vi "UPDATE FROM DB.vi"(8 "error in":errorcluster, 10 "object":refnum<class "_ISerializable.lvclass">, 11 "orm in":refnum<class "LV-ORM.lvclass">) -> (0 "error out":errorcluster, 3 "orm out":refnum<class "LV-ORM.lvclass">)   [LabVIEW 2018, in "LV-ORM.lvclass"]
uses:
  LV-ORM.lvclass
  _Serializable Base Object/_ISerializable.lvclass
  <userlib>/_OpenG.lib/array/array.llb/Filter 1D Array (String)__ogtk.vi
  <userlib>/_OpenG.lib/array/array.llb/Delete Elements from 1D Array (String)__ogtk.vi
  Serializer/Serializer.lvclass
panel:
  out "column names":string[](array[string])
  out "names":string[](array[string])
  out "recordset data":variant[][](array[variant])
  out "x != y?":bool[](array[boolean])
  out "update query":string
  out "select query":string
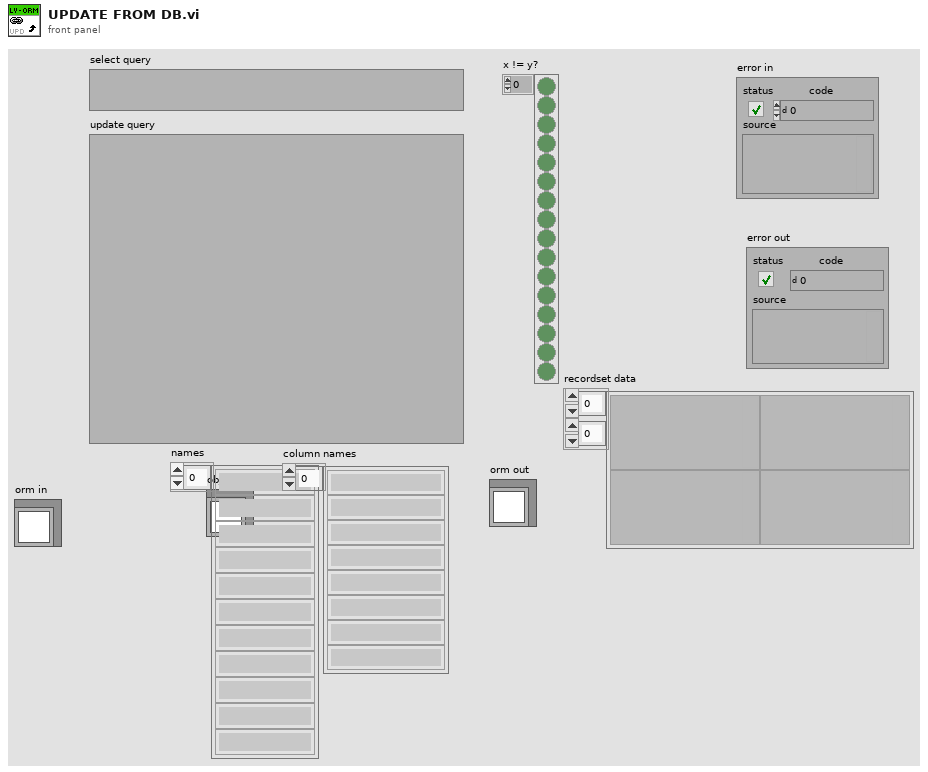
[diagram p1: front panel]
types:
  T1 = typedef "key-value-type cluster.ctl" = cluster{"names":string[], "values":string[], "type":string[], "class name":string}
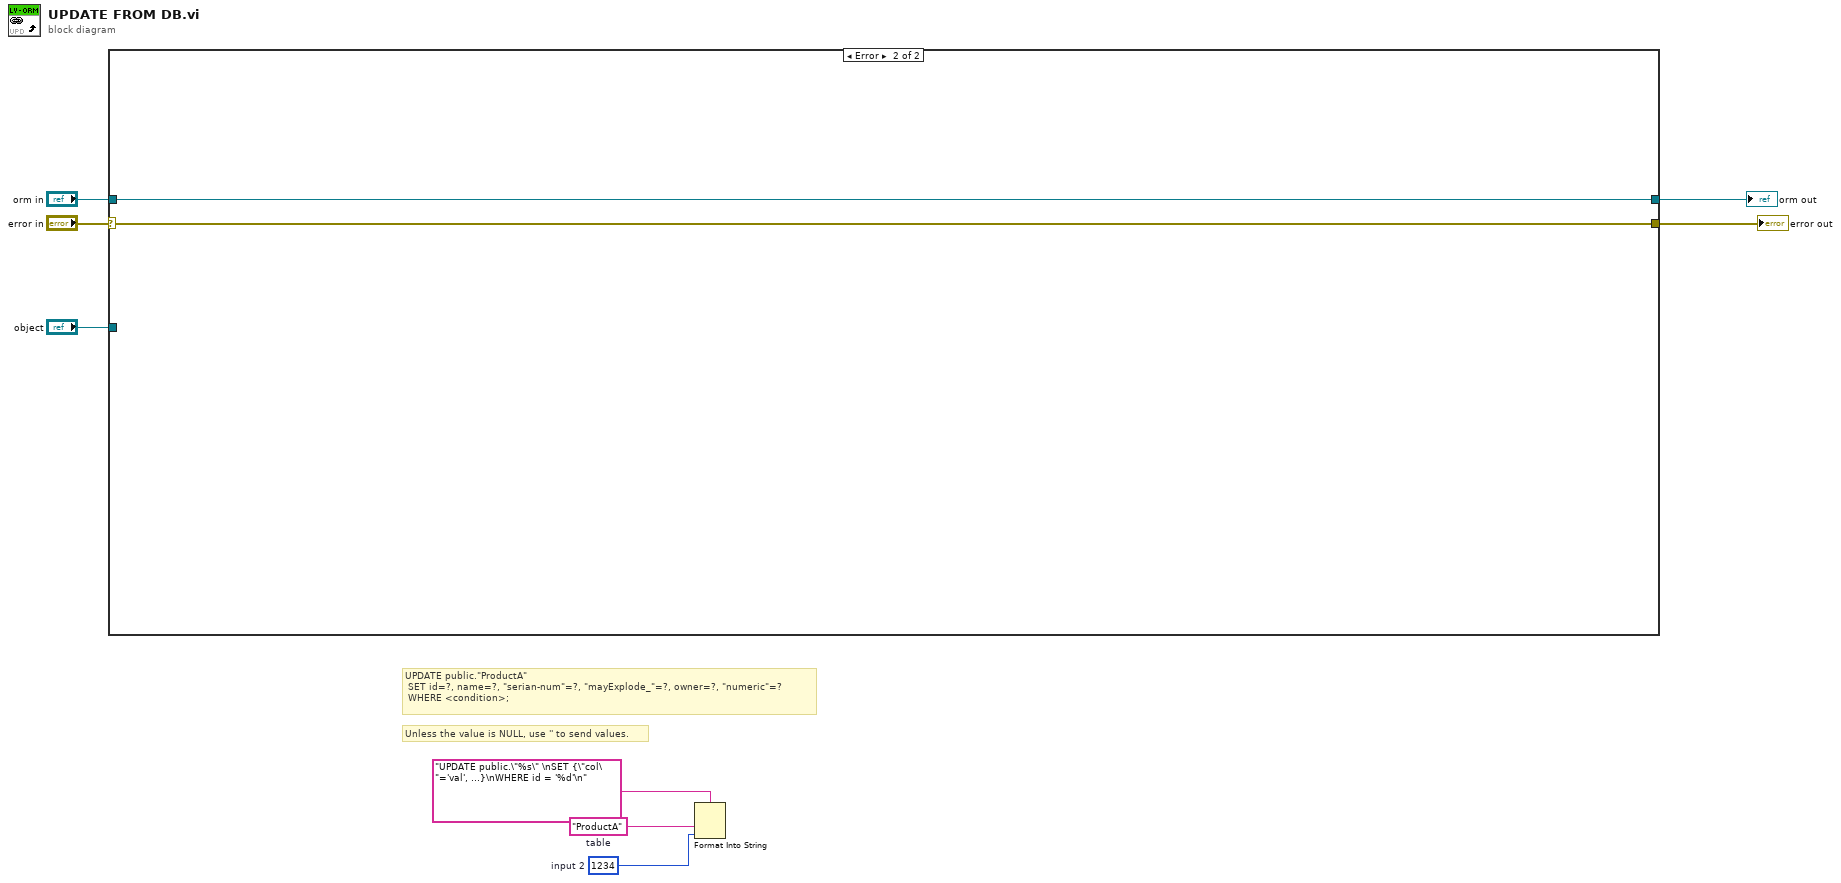
[diagram p0: block diagram]
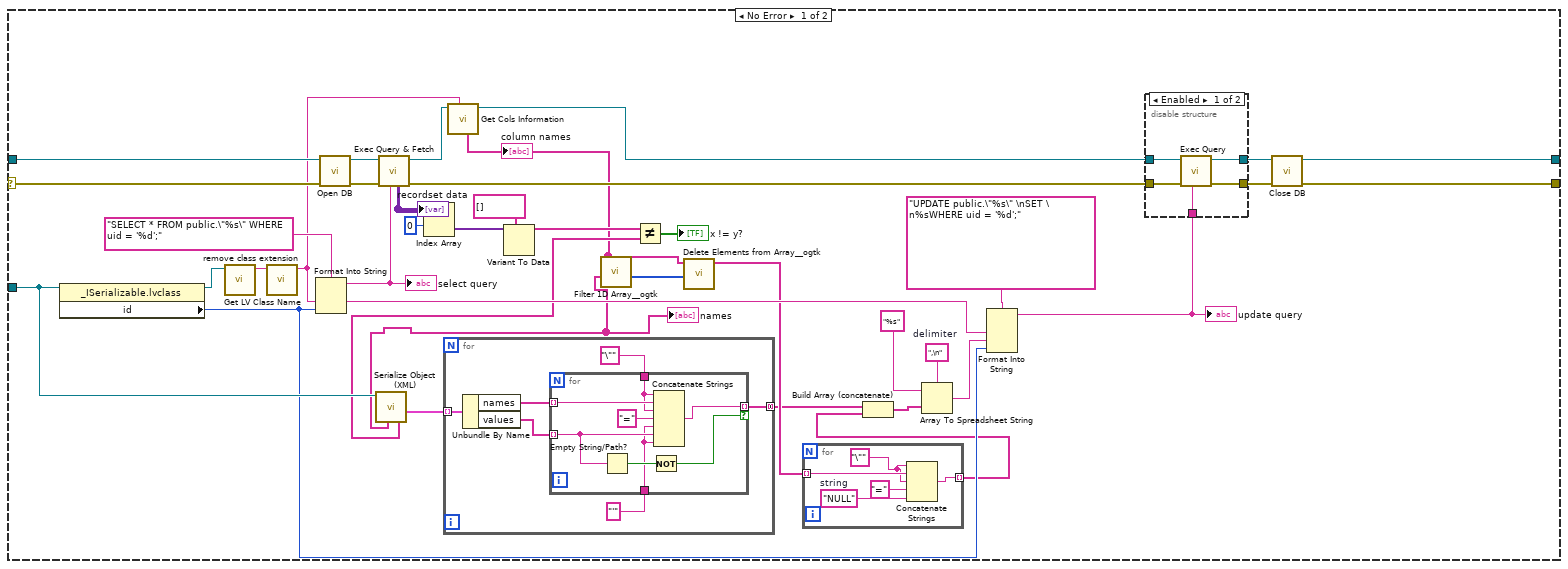
[diagram p2: hidden frame]
diagram:
  w1 = 1234  # input 2
  w2 = "ProductA"  # table
  # "Unless the value is NULL, use '' to send values."
  # "UPDATE public.\"ProductA\"\n\tSET id=?, name=?, \"serian-num\"=?, \"mayExplode_\"=?, owner=?, \"numeric\"=?\n\tWHERE <condition>;"
  n1 = case shown="Error" "error in" {
    selector: "error in" -> [w33 w74]
    tunnel: [w26 w74] -> w7
    tunnel: [w43 w73] -> w6
    tunnel: "orm in" -> [w42 w73]
    tunnel: "object" -> [w37 _]
    frame No Error {
      w30 = ",\n"  # delimiter
      n2 = property class="_ISerializable.lvclass"(reference=w37) -> (reference out=w39:refnum<class "_ISerializable.lvclass">, "id"=w27:i32)  [unwired: 1 in, 1 out]
      n3 = call <vilib>:"Get LV Class Name.vi"("object"=w39) -> ("class name"=w40:string)  [unwired: 9 in, 1 out]
      n4 = call "remove class extension.vi"("class name in"=w40) -> ("class name out"=w18:string)  [unwired: 10 in]
      n5 = Format Into String(format string="SELECT * FROM public.\"%s\" WHERE uid = '%d';", w18, w27) -> (resulting string=w13:string)  [unwired: 2 in, 1 out]
      "select query" <- w13
      n6 = call "Open DB.vi"("error in (no error)"=w33, "LV-ORM in"=w42) -> ("error out"=w38:errorcluster, "LV-ORM out"=w41:refnum<class "LV-ORM.lvclass">)  [unwired: 8 in]
      n7 = call "Serialize Object (XML).vi"("object in"=w37) -> ("key-value-type"=w29:T1[], "values"=w16:string[], "names"=w9:string[])  [unwired: 6 in, 2 out]
      "names" <- w9
      n8 = call "Exec Query & Fetch.vi"("scripts"=w13, "error in"=w38, "orm in"=w41) -> ("error out"=w34:errorcluster, "orm out"=w20:refnum<class "LV-ORM.lvclass">, "recordset data"=w36:variant[][])  [unwired: 6 in]
      "recordset data" <- w36
      n9 = Index Array(array=w36, index (row)=0) -> (element=w32:variant[])  [unwired: 1 in]
      n10 = for {
        tunnel: w29 -> [w57] mode=indexing
        tunnel: [w56] -> w12 mode=concatenating
        n11 = Unbundle By Name(w57) -> ("names"=w55:string[], "values"=w53:string[])
        n12 = for {
          tunnel: w55 -> [w65] mode=indexing
          tunnel: [w64] -> w56 mode=indexing if=w59
          tunnel: "\"" -> [w63]
          tunnel: w53 -> [w61] mode=indexing
          tunnel: "'" -> [w58]
          n13 = Empty String/Path?(string/path=w61) -> (empty?=w60:bool)
          n14 = Not(x=w60) -> (.not. x?=w59:bool)
          n15 = Concatenate Strings(w63, w65, w63, "=", w58, w61, w58) -> (w64:string)
        }
      }
      n16 = call "Get Cols Information.vi"("Table Name"=w18, "LV-ORM in"=w20) -> ("LV-ORM out"=w19:refnum<class "LV-ORM.lvclass">, "column names"=w15:string[])  [unwired: 5 in, 3 out]
      "column names" <- w15
      n17 = Variant To Data(type=string[] [], Variant=w32) -> (data=w22:string[])  [unwired: 1 in, 1 out]
      n18 = call-poly <userlib>:"Filter 1D Array__ogtk.vi"("items to filter"=w9, "array"=w15) -> ("filtered item indices"=w14:i32[])  [unwired: 4 in, 1 out]
      n19 = Not Equal?(x=w22, y=w16) -> (x != y?=→"x != y?":bool[])
      n20 = call-poly <userlib>:"Delete Elements from Array__ogtk.vi"("indices"=w14, "array"=w15) -> ("array w/ subset deleted"=w17:string[])  [unwired: 8 in, 1 out]
      n21 = for {
        tunnel: w17 -> [w51] mode=indexing
        tunnel: [w50] -> w21 mode=indexing
        w47 = "NULL"  # string
        w48 = "\""
        n22 = Concatenate Strings(w48, w51, w48, "=", w47) -> (w50:string)
      }
      n23 = Build Array (concatenate)(w12, w21) -> (w10:string[])
      n24 = Array To Spreadsheet String(delimiter (Tab)=w30, array=w10, 3:"%s") -> (spreadsheet string=w28:string)
      n25 = Format Into String(format string="UPDATE public.\"%s\" \nSET \n%sWHERE uid = '%d';", w18, w28, w27) -> (resulting string=w11:string)  [unwired: 2 in, 1 out]
      "update query" <- w11
      n26 = disable-structure shown="Enabled" {
        disable-tunnel: [w70 w72] -> w45
        disable-tunnel: [w69 w71] -> w44
        disable-tunnel: w19 -> [w68 w72]
        disable-tunnel: w34 -> [w66 w71]
        disable-tunnel: w11 -> [w67 _]
        frame Enabled {
          n27 = call "Exec Query.vi"("scripts"=w67, "error in"=w66, "orm in"=w68) -> ("error out"=w69:errorcluster, "orm out"=w70:refnum<class "LV-ORM.lvclass">)  [unwired: 7 in]
        }
        frame Disabled {
        }
      }
      n28 = call "Close DB.vi"("error in"=w44, "LV-ORM in"=w45) -> ("error out"=w26:errorcluster, "LV-ORM out"=w43:refnum<class "LV-ORM.lvclass">)  [unwired: 8 in]
    }
    frame Error {
    }
  }
  "error out" <- w7
  "orm out" <- w6
  n29 = Format Into String(format string="UPDATE public.\"%s\" \nSET {\"col\"='val', ...}\nWHERE id = '%d'\n", w2, w1) -> ()  [unwired: 2 in, 2 out]
